vi "Get Relay Names.vi"(8 "error in":errorcluster, 11 "2525 in":refnum<class "2525.lvclass">) -> (0 "error out":errorcluster, 3 "2525 out":refnum<class "2525.lvclass">)   [LabVIEW 2019, in "2525.lvlib" / "2525.lvclass"]
uses:
  Library/2525.lvclass
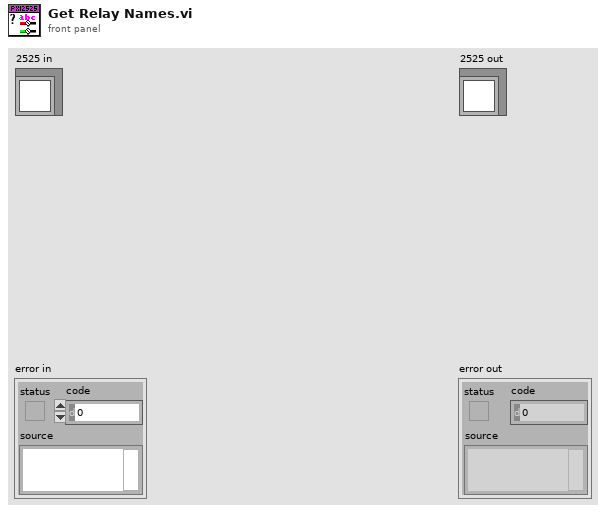
[diagram p1: front panel]
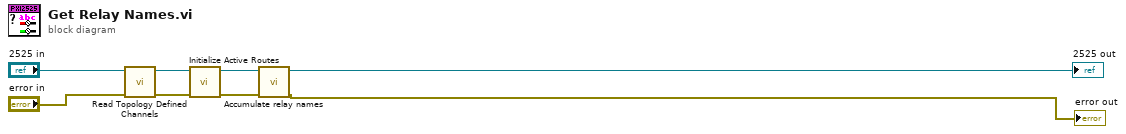
[diagram p0: block diagram]
diagram:
  n1 = call "Read Topology Defined Channels.vi"("error in"="error in", "2525 in"="2525 in") -> ("error out"=w6:errorcluster, "2525 out"=w5:refnum<class "2525.lvclass">)  [unwired: 8 in]
  n2 = call "Initialize Active Routes.vi"("error in (no error)"=w6, "2525 in"=w5) -> ("error out"=w4:errorcluster, "2525 out"=w3:refnum<class "2525.lvclass">)  [unwired: 8 in]
  n3 = call "Accumulate relay names.vi"("error in (no error)"=w4, "2525 in"=w3) -> ("error out"=→"error out":errorcluster, "2525 out"=→"2525 out":refnum<class "2525.lvclass">)  [unwired: 8 in]
